vi "toStringArray.vi"(8 "error in (no error)":errorcluster, 11 "RfRamp in":refnum<class "RfRamp.lvclass">) -> (0 "error out":errorcluster, 2 "eventStringArray":string[](array[string]), 3 "RfRamp out":refnum<class "RfRamp.lvclass">)   [LabVIEW 2009, in "Tools.lvlib" / "Scripting.lvlib" / "RfRamp.lvclass"]
uses:
  RfRamp.lvclass
  Rf Event/rf.lvclass
  RfRamp.lvclass/RfRamp.ctl
  ScriptEvent.lvclass
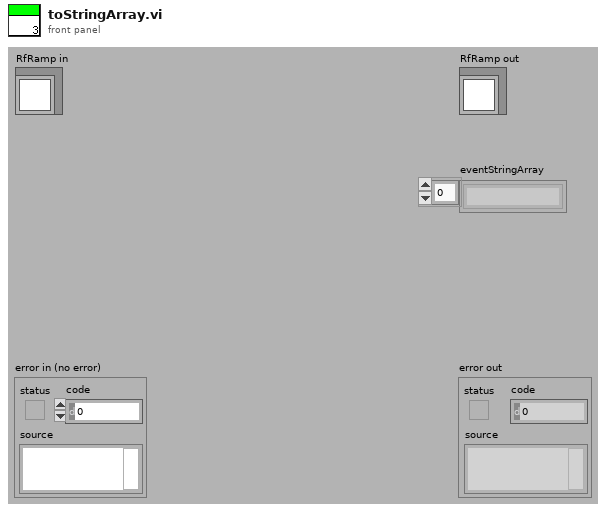
[diagram p1: front panel]
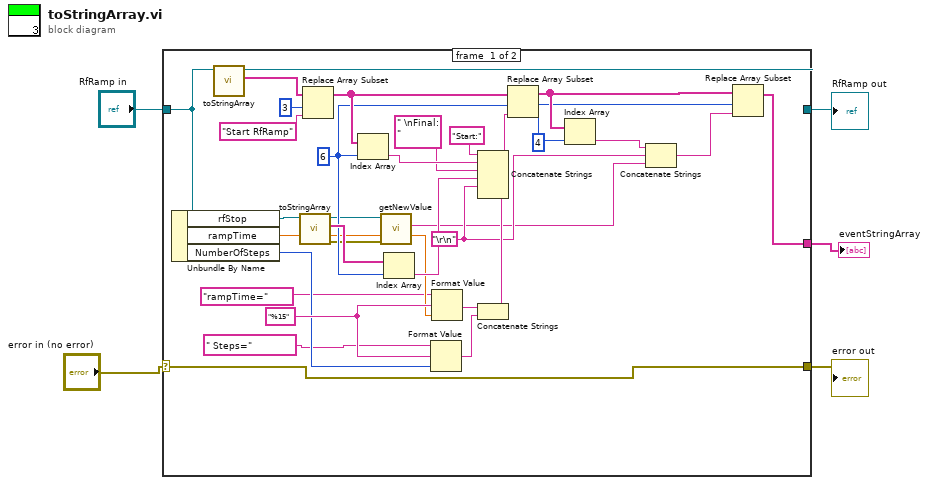
[diagram p0: block diagram]
diagram:
  n1 = case shown="No Error" "error in (no error)" {
    selector: "error in (no error)" -> [w37 w38]
    tunnel: [w37 w38] -> w4
    tunnel: [w24 w39] -> w3
    tunnel: "RfRamp in" -> [w36 w39]
    tunnel: [w6 _] -> w1
    frame #0 {
      w11 = 4
      w23 = "%15"
      w9 = "\r\n"
      w25 = 6
      n2 = Unbundle By Name(w36) -> ("rfStop"=w32:refnum<class "rf.lvclass">, "rampTime"=w21:dbl, "NumberOfSteps"=w20:i32)
      n3 = call-parent "toStringArray.vi"("rf in"=w36) -> ("eventStringArray"=w33:string[], "rf out"=w24:refnum<class "RfRamp.lvclass">)  [unwired: 8 in, 1 out]
      n4 = call-parent "toStringArray.vi"("rf in"=w32) -> ("error out"=w13:errorcluster, "eventStringArray"=w29:string[], "rf out"=w14:refnum<class "rf.lvclass">)  [unwired: 8 in]
      n5 = Replace Array Subset(array=w33, new element="Start RfRamp", index=3) -> (w27:string[])
      n6 = Index Array(array=w27, index=w25) -> (element=w31:string)
      n7 = call "getNewValue.vi"("error in (no error)"=w13, "ScriptEvent.lvclass in"=w14) -> ("newValue"=w8:string)  [unwired: 7 in, 2 out]
      n8 = Index Array(array=w29, index=w25) -> (element=w28:string)
      n9 = Format Value(string ("")=" Steps=", format string=w23, value (0)=w20) -> (output string=w22:string)
      n10 = Format Value(string ("")="rampTime=", format string=w23, value (0)=w21) -> (output string=w18:string)
      n11 = Concatenate Strings(w18, w22) -> (w17:string)
      n12 = Concatenate Strings("Start:", w31, " \nFinal: ", w28, w9, w17) -> (w26:string)
      n13 = Replace Array Subset(array=w27, new element=w26, index=w25) -> (w12:string[])
      n14 = Index Array(array=w12, index=w11) -> (element=w10:string)
      n15 = Concatenate Strings(w10, w9, w8) -> (w7:string)
      n16 = Replace Array Subset(array=w12, new element=w7, index=w11) -> (w6:string[])
    }
    frame #1 {
    }
  }
  "error out" <- w4
  "RfRamp out" <- w3
  "eventStringArray" <- w1
